vi "Get myRIO Image.vi"() -> ()   [LabVIEW 2014]
uses:
  <vilib>/nisyscfg/Software 1.2.ctl
  <vilib>/nisyscfg/Component Type.ctl
  <vilib>/nisyscfg/Create System Image (File).vi
  <vilib>/nisyscfg/nisyscfg.lvlib
panel:
  out "error out":errorcluster
  in  "Image Metadata in":T1={"title"="Robot Remote Control", "description"="This Image is of a myRIO for communicating using the CyberSim version 0.4", "ID"="", "version"="0.4", "component type"=5} {"component type" items=["standard", "hidden", "system", "unknown", "startup", "image"]}
  in  "Destination File":path
  in  "Session in":refnum<k21>
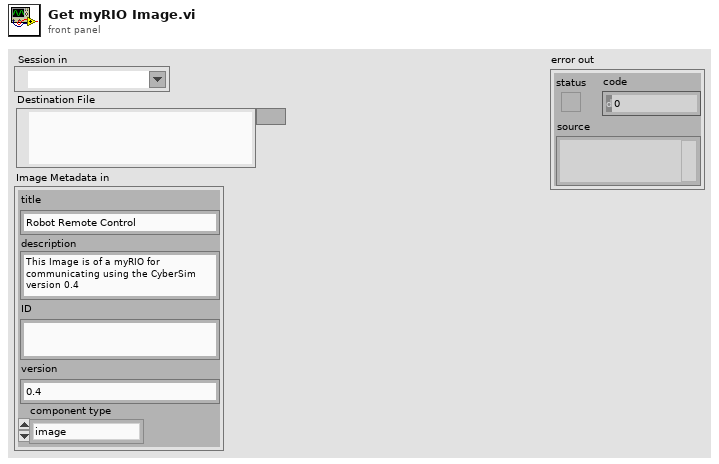
[diagram p1: front panel]
types:
  T1 = typedef "nisyscfg.lvlib/Software 1.2.ctl" = cluster{"title":string, "description":string, "ID":string, "version":string, "component type":T2}
  T2 = typedef "nisyscfg.lvlib/Component Type.ctl" = u32
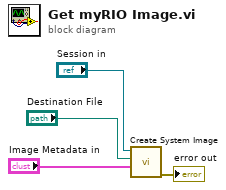
[diagram p0: block diagram]
diagram:
  n1 = call-poly <vilib>:"Create System Image.vi"("Image Metadata in"="Image Metadata in", "Destination File"="Destination File", "Session in"="Session in") -> ("error out"=→"error out":errorcluster)  [unwired: 6 in, 2 out]
